vi "logCase.vi"(11 "CaseControl.histCase":T2(array[cluster])) -> (3 "oper":string)   [LabVIEW 2018]
uses:
  TEST/Typedefs/Command.ctl
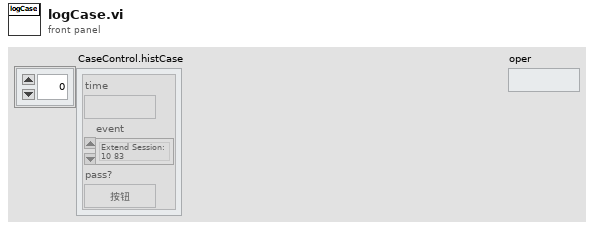
[diagram p1: front panel]
types:
  T1 = typedef "Command.ctl" = enum16{"Extend Session: 10 83", "Tester Present: 3E 80", "Resquest Seed: 27 01", "Send Key: 27 02", "Check FBL:  31 01 FD 02", "Control DTC: 85 82", "Comm Control: 28 83 01", "Program Session Request: 10 02", "Request Seed: 27 35", "Seed Key: 27 36", "Request Download: 34 00 44", "Transfer Data: 36 XX YY", "More Data?", "Request Transfer Exit: 37", "Check Flash Driver Validity: 01 FD 03", "More Segment?", "Write Data Fingereint: 23 F1 F0+26", "EraseFlashMemory Routine: 31 01 FD 00 44", "More segment?(each file)", "CheckAppSwAppData Validity: 31 01 FD 04 44", "CheckAppSwAppData Dependency: 31 01 fd 01", "ECU Reset: 11 81", "System: Init", "System: Idle", "System: Error", "System: Wait", "System: Delay", "System: CAN Send", "System: Exit"}
  T2 = cluster{"time":string, "event":T1, "pass?":bool}[]
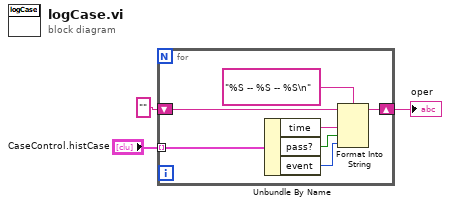
[diagram p0: block diagram]
diagram:
  n1 = for {
    tunnel: "CaseControl.histCase" -> [w10] mode=indexing
    shift-right: [w6] -> w2
    shift-left: "" -> [w5]
    n2 = Unbundle By Name(w10) -> ("time"=w8:string, "pass?"=w9:bool, "event"=w4:T1)
    n3 = Format Into String(format string="%S -- %S -- %S\n" ("格式字符串"), initial string=w5, w8, w9, w4) -> (resulting string=w6:string)  [unwired: 1 in, 1 out]
  }
  "oper" <- w2
